vi "DetectFreezeFinal.vi"(8 "error in (no error)":errorcluster, 11 "Droplets Proccesed":refnum<vi>) -> (0 "error out":errorcluster)   [LabVIEW 2013]
doc: "Use this template to build a VI to use as a subVI."
uses:
  DB/DbEnum.ctl
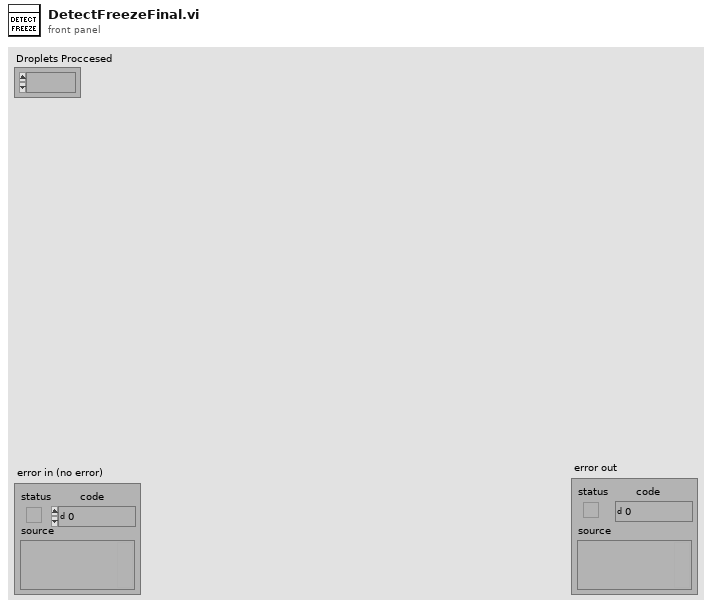
[diagram p1: front panel]
types:
  T1 = typedef "DbEnum.ctl" = enum16{"Write DropletDB", "Init", "Insert Detection Result Data", "Insert Grey Level Result", "Insert Baseline Results", "AddFreezeImagesAtCertainDroplet", "UpdateIncludeDroplet", "Insert Freeze Analysis Results", "GetDropDB", "GetNoFreezedDroplets", "GetGreyLevelAndDiff", "GetGreyLevelatIndexTime", "GetDropletsBoundingBox"}
  T2 = cluster{"ImageIndexArray":u32[], "GreyLevelInBoundingBox":dbl[][], "GLDifference":dbl[][]}
  T3 = typedef "FreezePointData.ctl" = cluster{"Freeze YesNo":cluster{"Freeze Grey Diff value":dbl, "Freeze Point Found":bool, "Freeze Indices":u32[]}[], "Rel Time":u32[]}
  T4 = cluster{"DropletBaseline":dbl[], "DropletBaselineSTD":dbl[]}
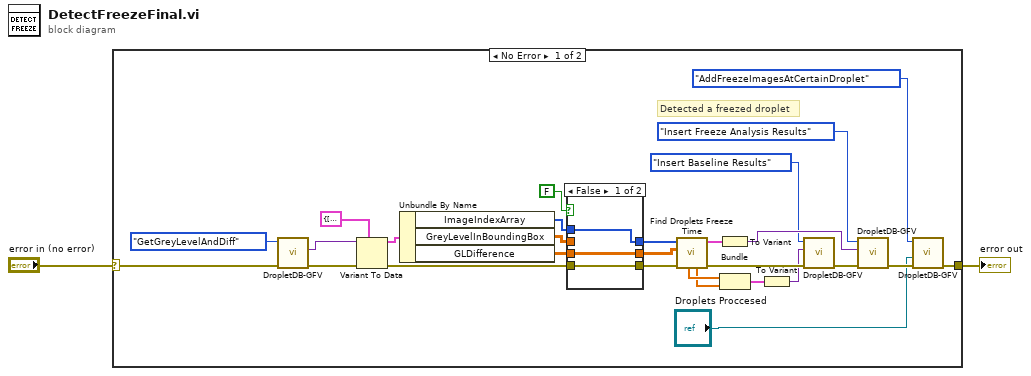
[diagram p0: block diagram]
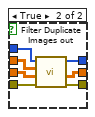
[diagram p2: hidden frame]
diagram:
  n1 = case shown="No Error" "error in (no error)" {
    selector: "error in (no error)" -> [w18 w41]
    tunnel: [w17 w41] -> w1
    frame No Error {
      # "Detected a freezed droplet"
      n2 = call "DropletDB-GFV.vi"("error in (no error)"=w18, "Command In"=DbEnum."GetGreyLevelAndDiff") -> ("error out"=w30:errorcluster, "Data out"=w29:variant)  [unwired: 8 in]
      n3 = Variant To Data(error in=w30, type=T2 {"ImageIndexArray"=[], "GreyLevelInBoundingBox"=[], "GLDifference"=[]} ("output cluster"), Variant=w29) -> (data=w27:T2, error out=w25:errorcluster)
      n4 = Unbundle By Name(w27) -> ("ImageIndexArray"=w5:u32[], "GreyLevelInBoundingBox"=w26:dbl[][], "GLDifference"=w4:dbl[][])
      n5 = case shown="False" FALSE {
        tunnel: w5 -> [w33 w40]
        tunnel: w26 -> [_ w39]
        tunnel: w4 -> [w32 w38]
        tunnel: w25 -> [w31 w37]
        tunnel: [w32 w36] -> w6
        tunnel: [w31 w35] -> w24
        tunnel: [w33 w34] -> w7
        frame False {
        }
        frame True {
          n6 = call "Filter Duplicate Images out.vi"("Error In"=w37, "GreyLevel Drops and time Derivative in"=w38, "GreyLevel Drops and time in"=w39, "Rel Time (s) in"=w40) -> ("Error Out"=w35:errorcluster, "GreyLevel Drops and time Derivative out"=w36:dbl[][], "Rel Time (s) out"=w34:u32[])  [unwired: 4 in, 1 out]
        }
      }
      n7 = call "Find Droplets Freeze Time.vi"("Error In"=w24, "GreyLevel Drops and time Derivative in"=w6, "Rel Time Array"=w7) -> ("Error Out"=w23:errorcluster, "FreezeYesNo"=w20:T3, "DropletBaselineSTD"=w21:dbl[], "DropletBaseline"=w22:dbl[])  [unwired: 5 in]
      n8 = To Variant(anything=w20) -> (Variant=w15:variant)
      n9 = Bundle("DropletBaseline"=w22, "DropletBaselineSTD"=w21) -> (w10:T4)  [unwired: 1 in]
      n10 = To Variant(anything=w10) -> (Variant=w9:variant)
      n11 = call "DropletDB-GFV.vi"("error in (no error)"=w23, "Data in"=w9, "Command In"=DbEnum."Insert Baseline Results") -> ("error out"=w8:errorcluster)  [unwired: 7 in, 1 out]
      n12 = call "DropletDB-GFV.vi"("error in (no error)"=w8, "Data in"=w15, "Command In"=DbEnum."Insert Freeze Analysis Results") -> ("error out"=w12:errorcluster)  [unwired: 7 in, 1 out]
      n13 = call "DropletDB-GFV.vi"("error in (no error)"=w12, "Droplets Proccesed"="Droplets Proccesed", "Command In"=DbEnum."AddFreezeImagesAtCertainDroplet") -> ("error out"=w17:errorcluster)  [unwired: 7 in, 1 out]
    }
    frame Error {
    }
  }
  "error out" <- w1
